vi "compteur.vi"() -> ()   [LabVIEW 2020]
panel:
  out "compteur":dbl
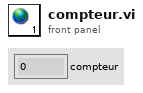
[diagram p1: front panel]
diagram:
